vi "Write Shell hwnd .vi"(8 "error in (no error)":errorcluster, 10 "Shell hwnd":u32=921718, 11 "Py Doc in":refnum<class "Py Doc.lvclass">) -> (0 "error out":errorcluster, 3 "Py Doc out":refnum<class "Py Doc.lvclass">)   [LabVIEW 2016, in "Py Doc.lvclass"]
uses:
  Py Doc.lvclass
  Py Doc.lvclass/Py Doc.ctl
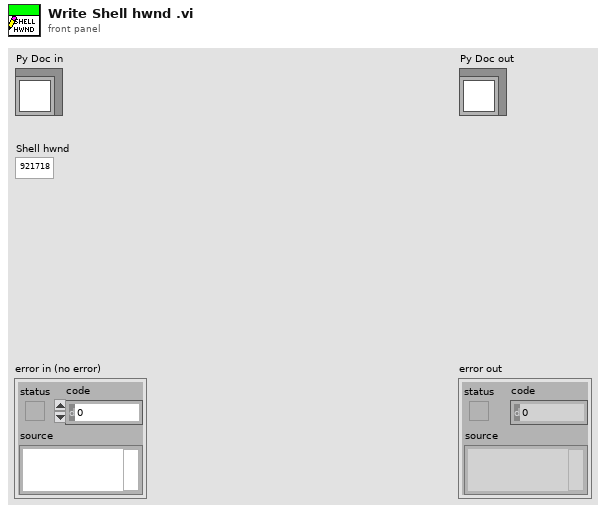
[diagram p1: front panel]
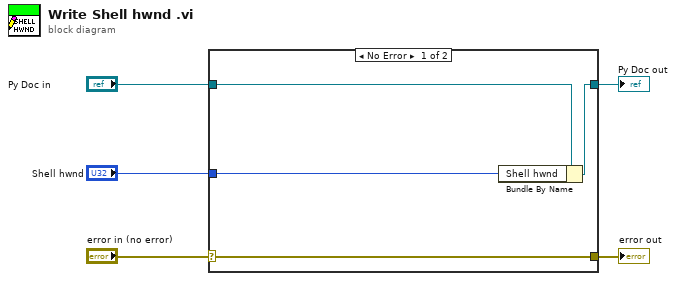
[diagram p0: block diagram]
diagram:
  n1 = case shown="No Error" "error in (no error)" {
    selector: "error in (no error)" -> [w9 w10]
    tunnel: [w9 w10] -> w4
    tunnel: [w7 w11] -> w2
    tunnel: "Py Doc in" -> [w8 w11]
    tunnel: "Shell hwnd" -> [w6 _]
    frame No Error {
      n2 = Bundle By Name(cluster=w8, "Shell hwnd"=w6) -> (w7:refnum<class "Py Doc.lvclass">)
    }
    frame Error {
    }
  }
  "error out" <- w4
  "Py Doc out" <- w2
